vi "Stoerungen (321-384) - VFS3.vi"(8 "Fehler (Eingang)":errorcluster caption="Fehler (Eingang, kein Fehler)") -> (0 "Fehler (Ausgang)":errorcluster, 3 "Störungen 321-384":u64)   [LabVIEW 2015, in "Stoerungen.lvlib"]
uses:
  Stoerungen.lvlib
  PNS/Parameternamen PNS.ctl
  PNS/PNS.lvlib
  Stoerungen Messgeraet/Aktionen Kommunikation Stoerung.ctl
  Seiten/System Einstellungen/System Einstellungen.lvlib
  Seiten/System Einstellungen/Aktioen FGV System.ctl
  PNS/Aktionen FGV Istwerte.ctl
  cRIO/Stoermeldungen/Stoerungen 321-384.ctl
  cRIO/Stoermeldungen/Stoermeldungen.lvlib
panel:
  # "Störmeldungen PNS (321-384)"
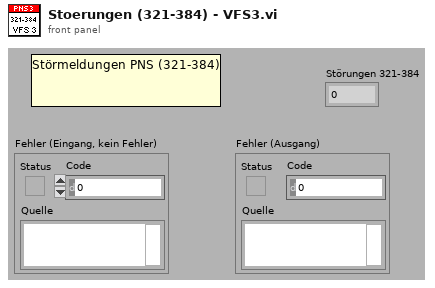
[diagram p1: front panel]
types:
  T1 = typedef "System Einstellungen.lvlib/Aktioen FGV System.ctl" = enum16{"lesen", "laden", "speichern", "Optionen schreiben", "Zeitstempel", "Reset BMP", "Reset SQP", "Wartung"}
  T2 = typedef "System Einstellungen.lvlib/Optionen.ctl" = cluster{"Störmeldep.":bool, "Betriebszustände":bool, "LN2 Befüllung":bool, "Klimaanlage ?":bool, "AK in ppm":bool, "log Cal-Gas":bool, "log 0-Gas":bool, "log CG zu PNS":bool, "Reserve":bool, "Reserve1":bool, "PNS?":bool, "Container":bool, "Mit N2 spülen":bool, "Span Gas Auswahl":T3, "VFS 1":bool, "VFS 2":bool, "VFS 3":bool, "VFS 4":bool, "TRE08":bool}
  T3 = typedef "Funktionstasten.lvlib/Spaneingang.ctl" = u16
  T4 = typedef "PNS.lvlib/Parameternamen PNS.ctl" = enum16{"Heizkreis 1", "Heizkreis 2", "Heizkreis 3", "Heizkreis 4", "Heizkreis 5", "Heizkreis 6", "Heizkreis 7", "Heizkreis 8"}
  T5 = typedef "PNS.lvlib/Aktionen FGV Istwerte.ctl" = enum16{"lesen", "initialisieren", "schreiben", "Störungen"}
  T6 = typedef "Stoerungen.lvlib/Aktionen Kommunikation Stoerung.ctl" = enum16{"lesen", "init", "FT-IR Komm", "FT-IR Betriebsart", "FT-IR Hintergrund", "cRIO Komm", "PNS Komm", "Dichtheitstest", "Life Bit", "FTIR Komm AK", "PMA Komm", "FID Komm", "PMA Cal", "FID Ch4 Cal", "FID THC Cal", "Cal Timeout", "VFS 1 Komm", "VFS 2 Komm", "VFS 3 Komm", "VFS 4 Komm", "TRE 08 Komm", "CG-Test vorzeitig", "CG-Test Span 1", "CG-Test Span 2", "CG-Test Span 3", "CG-Test Messgas", "CG-Test löschen", "Test", "Amium AK"}
  T7 = typedef "Stoermeldungen.lvlib/Stoerungen 321-384.ctl" = cluster{"ERR. 321":bool, "ERR. 322":bool, "ERR. 323":bool, "ERR. 324":bool, "ERR. 325":bool, "ERR. 326":bool, "ERR. 327":bool, "ERR. 328":bool, "ERR. 329":bool, "ERR. 330":bool, "ERR. 331":bool, "ERR. 332":bool, "ERR. 333":bool, "ERR. 334":bool, "ERR. 335":bool, "ERR. 336":bool, "ERR. 337":bool, "ERR. 338":bool, "ERR. 339":bool, "ERR. 340":bool, "ERR. 341":bool, "ERR. 342":bool, "ERR. 343":bool, "ERR. 344":bool, "ERR. 345":bool, "ERR. 346":bool, "ERR. 347":bool, "ERR. 348":bool, "ERR. 349":bool, "ERR. 350":bool, "ERR. 351":bool, "ERR. 352":bool, "ERR. 353":bool, "ERR. 354":bool, "ERR. 355":bool, "ERR. 356":bool, "ERR. 357":bool, "ERR. 358":bool, "ERR. 359":bool, "ERR. 360":bool, "ERR. 361":bool, "ERR. 362":bool, "ERR. 363":bool, "ERR. 364":bool, "ERR. 365":bool, "ERR. 366":bool, "ERR. 367":bool, "ERR. 368":bool, "ERR. 369":bool, "ERR. 370":bool, "ERR. 371":bool, "ERR. 372":bool, "ERR. 373":bool, "ERR. 374":bool, "ERR. 375":bool, "ERR. 376":bool, "ERR. 377":bool, "ERR. 378":bool, "ERR. 379":bool, "ERR. 380":bool, "ERR. 381":bool, "ERR. 382":bool, "ERR. 383":bool, "ERR. 384":bool}
  T8 = typedef "Steuerung PNS.lvclass/Regler.ctl" = cluster{"Istwert":i16, "Sollwert":i16, "Alarm MIN":i16, "Alarm MAX":i16, "Regler sperren":i16, "Analog Ausgang":i16}[]
  T9 = cluster{"Istwert":i16, "Sollwert":i16, "Alarm MIN":i16, "Alarm MAX":i16, "Regler sperren":i16, "Analog Ausgang":i16}
  T10 = typedef "Stoerungen.lvlib/Stoerungen Messgeraete.ctl" = cluster{"FT-IR Komm":bool, "FT-IR Betriebsart":bool, "FT-IR Hintergrundscan":bool, "Dichtheitstest":bool, "cRIO Komm":bool, "PNS Komm":bool, "Life Bit":bool, "FT-IR AK Komm":bool, "PMA Komm":bool, "FID Komm":bool, "PMA Cal":bool, "FID CH4 Cal":bool, "FID THC Cal":bool, "Cal Timeout":bool, "VFS 1 Komm":bool, "VFS 2 Komm":bool, "VFS 3 Komm":bool, "VFS 4 Komm":bool, "TRE 08 Komm":bool, "CG-Test":bool, "CG-Test 1":bool, "CG-Test 2":bool, "CG-Test 3":bool, "Messgas - Eingang":bool, "Amium AK Komm":bool}
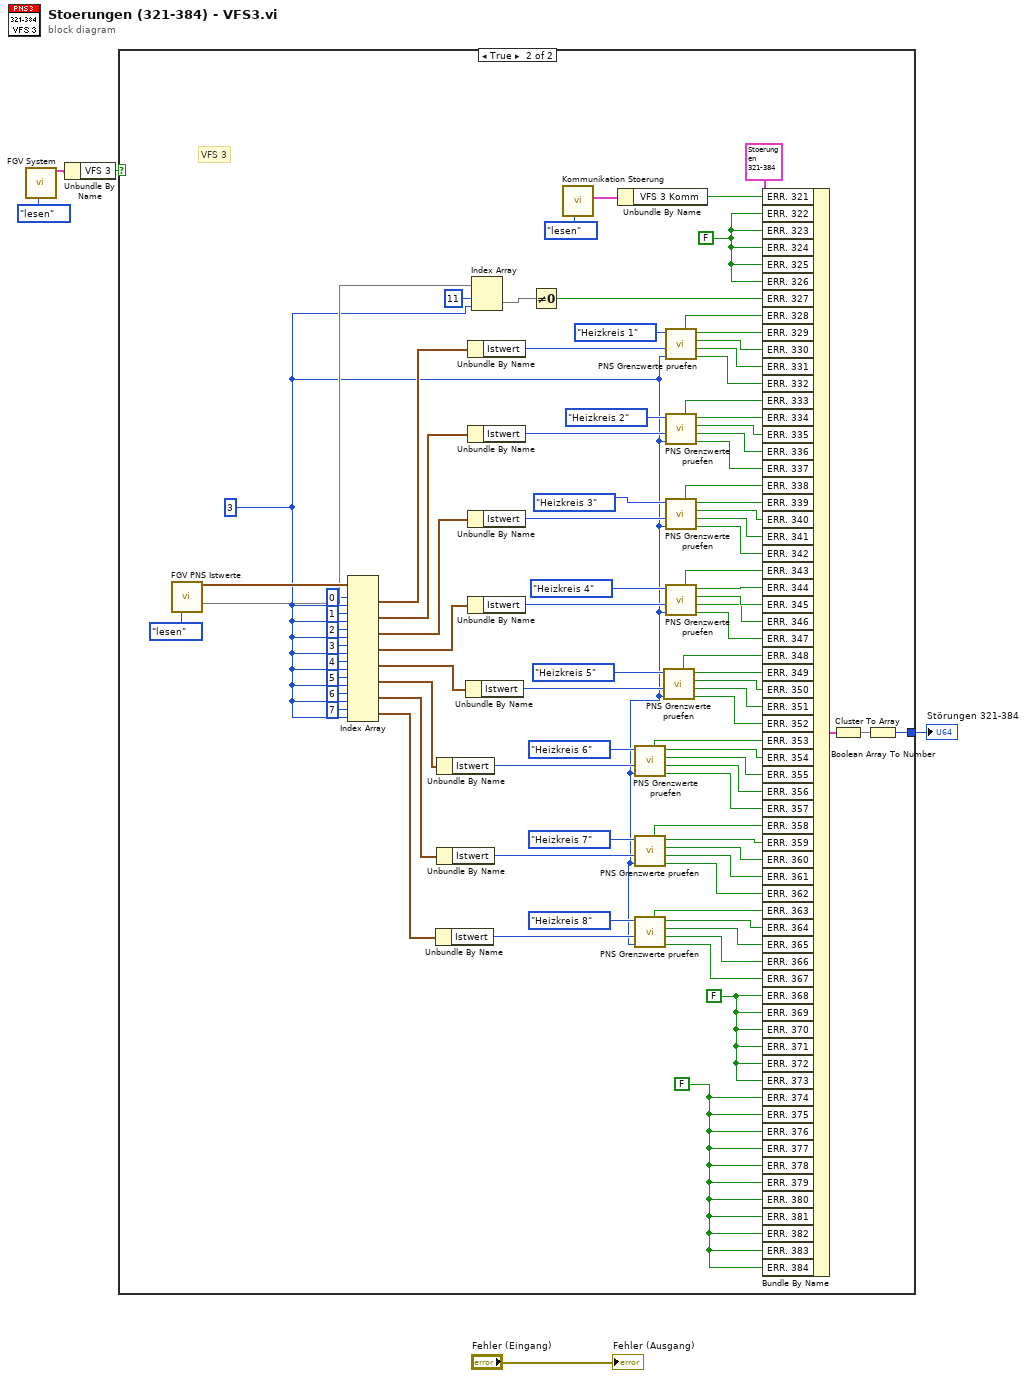
[diagram p0: block diagram]
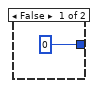
[diagram p2: hidden frame]
diagram:
  n1 = call "FGV System.vi"("Aktionen"=Aktioen_FGV_System."lesen") -> ("Optionen"=w3:T2)  [unwired: 13 in, 5 out]
  n2 = Unbundle By Name(w3) -> ("VFS 3"=w1:bool)
  n3 = case shown="True" w1 {
    tunnel: [u64 0 w55] -> w4
    frame False {
    }
    frame True {
      w7 = 3 ("Deaktivierter Index (Spalte)")
      w54 = FALSE ("ERR. 240")
      w62 = FALSE ("ERR. 194")
      w60 = FALSE ("ERR. 194")
      # "VFS 3"
      n4 = call "FGV PNS Istwerte.vi"("Aktionen"=Aktionen_FGV_Istwerte."lesen") -> ("Regler"=w92:T8, 10:w59)  [unwired: 10 in, 3 out]
      n5 = Index Array(array=w92, index (row) #1=0 ("Deaktivierter Index (Zeile)"), index (col) #1=w7, index (row) #2=1 ("Deaktivierter Index (Zeile)"), index (col) #2=w7, index (row) #3=2 ("Deaktivierter Index (Zeile)"), index (col) #3=w7, index (row) #4=3 ("Deaktivierter Index (Zeile)"), index (col) #4=w7, index (row) #5=4 ("Deaktivierter Index (Zeile)"), index (col) #5=w7, index (row) #6=5 ("Deaktivierter Index (Zeile)"), index (col) #6=w7, index (row) #7=6 ("Deaktivierter Index (Zeile)"), index (col) #7=w7, index (row) #8=7 ("Deaktivierter Index (Zeile)"), index (col) #8=w7) -> (element #1=w91:T9, element #2=w89:T9, element #3=w88:T9, element #4=w87:T9, element #5=w48:T9, element #6=w42:T9, element #7=w41:T9, element #8=w40:T9)
      n6 = Unbundle By Name(w40) -> ("Istwert"=w19:i16)
      n7 = Unbundle By Name(w42) -> ("Istwert"=w20:i16)
      n8 = Unbundle By Name(w41) -> ("Istwert"=w21:i16)
      n9 = Unbundle By Name(w48) -> ("Istwert"=w17:i16)
      n10 = Unbundle By Name(w91) -> ("Istwert"=w90:i16)
      n11 = Unbundle By Name(w89) -> ("Istwert"=w51:i16)
      n12 = Unbundle By Name(w88) -> ("Istwert"=w86:i16)
      n13 = Unbundle By Name(w87) -> ("Istwert"=w85:i16)
      n14 = Index Array(array=w59, index (row)=11 ("Index"), index (col)=w7) -> (element=w57)
      n15 = Not Equal To 0?(x=w57) -> (x != 0?=w56:bool)
      n16 = call "Kommunikation Stoerung.vi"("Aktionen"=Aktionen_Kommunikation_Stoerung."lesen") -> ("Störung Messgerät"=w64:T10)  [unwired: 10 in]
      n17 = Unbundle By Name(w64) -> ("VFS 3 Komm"=w61:bool)
      n18 = call "PNS Grenzwerte pruefen.vi"("Option"=w7, "Wert"=w20, "Parameternamen PNS"=Parameternamen_PNS."Heizkreis 6") -> ("AbschMax"=w35:bool, "AbschMin"=w36:bool, "WarnMax"=w37:bool, "WarnMin"=w38:bool, "F.Br."=w39:bool)  [unwired: 4 in]
      n19 = call "PNS Grenzwerte pruefen.vi"("Option"=w7, "Wert"=w21, "Parameternamen PNS"=Parameternamen_PNS."Heizkreis 7") -> ("AbschMax"=w30:bool, "AbschMin"=w31:bool, "WarnMax"=w32:bool, "WarnMin"=w33:bool, "F.Br."=w34:bool)  [unwired: 4 in]
      n20 = call "PNS Grenzwerte pruefen.vi"("Option"=w7, "Wert"=w19, "Parameternamen PNS"=Parameternamen_PNS."Heizkreis 8") -> ("AbschMax"=w25:bool, "AbschMin"=w26:bool, "WarnMax"=w27:bool, "WarnMin"=w28:bool, "F.Br."=w29:bool)  [unwired: 4 in]
      n21 = call "PNS Grenzwerte pruefen.vi"("Option"=w7, "Wert"=w17, "Parameternamen PNS"=Parameternamen_PNS."Heizkreis 5") -> ("AbschMax"=w43:bool, "AbschMin"=w44:bool, "WarnMax"=w45:bool, "WarnMin"=w46:bool, "F.Br."=w47:bool)  [unwired: 4 in]
      n22 = call "PNS Grenzwerte pruefen.vi"("Option"=w7, "Wert"=w90, "Parameternamen PNS"=Parameternamen_PNS."Heizkreis 1") -> ("AbschMax"=w80:bool, "AbschMin"=w81:bool, "WarnMax"=w82:bool, "WarnMin"=w83:bool, "F.Br."=w84:bool)  [unwired: 4 in]
      n23 = call "PNS Grenzwerte pruefen.vi"("Option"=w7, "Wert"=w51, "Parameternamen PNS"=Parameternamen_PNS."Heizkreis 2") -> ("AbschMax"=w75:bool, "AbschMin"=w76:bool, "WarnMax"=w77:bool, "WarnMin"=w78:bool, "F.Br."=w79:bool)  [unwired: 4 in]
      n24 = call "PNS Grenzwerte pruefen.vi"("Option"=w7, "Wert"=w86, "Parameternamen PNS"=Parameternamen_PNS."Heizkreis 3") -> ("AbschMax"=w70:bool, "AbschMin"=w71:bool, "WarnMax"=w72:bool, "WarnMin"=w73:bool, "F.Br."=w74:bool)  [unwired: 4 in]
      n25 = call "PNS Grenzwerte pruefen.vi"("Option"=w7, "Wert"=w85, "Parameternamen PNS"=Parameternamen_PNS."Heizkreis 4") -> ("AbschMax"=w65:bool, "AbschMin"=w66:bool, "WarnMax"=w67:bool, "WarnMin"=w68:bool, "F.Br."=w69:bool)  [unwired: 4 in]
      n26 = Bundle By Name(cluster=T7 {"ERR. 321"=FALSE, "ERR. 322"=FALSE, "ERR. 323"=FALSE, "ERR. 324"=FALSE, "ERR. 325"=FALSE, "ERR. 326"=FALSE, "ERR. 327"=FALSE, "ERR. 328"=FALSE, "ERR. 329"=FALSE, "ERR. 330"=FALSE, "ERR. 331"=FALSE, "ERR. 332"=FALSE, "ERR. 333"=FALSE, "ERR. 334"=FALSE, "ERR. 335"=FALSE, "ERR. 336"=FALSE, "ERR. 337"=FALSE, "ERR. 338"=FALSE, "ERR. 339"=FALSE, "ERR. 340"=FALSE, "ERR. 341"=FALSE, "ERR. 342"=FALSE, "ERR. 343"=FALSE, "ERR. 344"=FALSE, "ERR. 345"=FALSE, "ERR. 346"=FALSE, "ERR. 347"=FALSE, "ERR. 348"=FALSE, "ERR. 349"=FALSE, "ERR. 350"=FALSE, "ERR. 351"=FALSE, "ERR. 352"=FALSE, "ERR. 353"=FALSE, "ERR. 354"=FALSE, "ERR. 355"=FALSE, "ERR. 356"=FALSE, "ERR. 357"=FALSE, "ERR. 358"=FALSE, "ERR. 359"=FALSE, "ERR. 360"=FALSE, "ERR. 361"=FALSE, "ERR. 362"=FALSE, "ERR. 363"=FALSE, "ERR. 364"=FALSE, "ERR. 365"=FALSE, "ERR. 366"=FALSE, "ERR. 367"=FALSE, "ERR. 368"=FALSE, "ERR. 369"=FALSE, "ERR. 370"=FALSE, "ERR. 371"=FALSE, "ERR. 372"=FALSE, "ERR. 373"=FALSE, "ERR. 374"=FALSE, "ERR. 375"=FALSE, "ERR. 376"=FALSE, "ERR. 377"=FALSE, "ERR. 378"=FALSE, "ERR. 379"=FALSE, "ERR. 380"=FALSE, "ERR. 381"=FALSE, "ERR. 382"=FALSE, "ERR. 383"=FALSE, "ERR. 384"=FALSE} ("STÖRUNGEN 193-256"), "ERR. 321"=w61, "ERR. 322"=w60, "ERR. 323"=w60, "ERR. 324"=w60, "ERR. 325"=w60, "ERR. 326"=w60, "ERR. 327"=w56, "ERR. 328"=w84, "ERR. 329"=w83, "ERR. 330"=w82, "ERR. 331"=w81, "ERR. 332"=w80, "ERR. 333"=w79, "ERR. 334"=w78, "ERR. 335"=w77, "ERR. 336"=w76, "ERR. 337"=w75, "ERR. 338"=w74, "ERR. 339"=w73, "ERR. 340"=w72, "ERR. 341"=w71, "ERR. 342"=w70, "ERR. 343"=w69, "ERR. 344"=w68, "ERR. 345"=w67, "ERR. 346"=w66, "ERR. 347"=w65, "ERR. 348"=w47, "ERR. 349"=w46, "ERR. 350"=w45, "ERR. 351"=w44, "ERR. 352"=w43, "ERR. 353"=w39, "ERR. 354"=w38, "ERR. 355"=w37, "ERR. 356"=w36, "ERR. 357"=w35, "ERR. 358"=w34, "ERR. 359"=w33, "ERR. 360"=w32, "ERR. 361"=w31, "ERR. 362"=w30, "ERR. 363"=w29, "ERR. 364"=w28, "ERR. 365"=w27, "ERR. 366"=w26, "ERR. 367"=w25, "ERR. 368"=w54, "ERR. 369"=w54, "ERR. 370"=w54, "ERR. 371"=w54, "ERR. 372"=w54, "ERR. 373"=w54, "ERR. 374"=w62, "ERR. 375"=w62, "ERR. 376"=w62, "ERR. 377"=w62, "ERR. 378"=w62, "ERR. 379"=w62, "ERR. 380"=w62, "ERR. 381"=w62, "ERR. 382"=w62, "ERR. 383"=w62, "ERR. 384"=w62) -> (w95:T7)
      n27 = Cluster To Array(cluster=w95) -> (array=w94:bool[])
      n28 = Boolean Array To Number ("Boolesches Array nach Zahl")(Boolean array=w94) -> (number=w55:u64)
    }
  }
  "Störungen 321-384" <- w4
  "Fehler (Ausgang)" <- "Fehler (Eingang)"
